vi "ActionVIOnCompile.vi"(8 "error in (no error)":errorcluster, 11 "Device Item Ref in":T1 format="%.0x") -> (0 "error out":errorcluster)   [LabVIEW 2015, in "Waveform-Processing-Custom-Device System Explorer.lvlib"]
uses:
  Waveform-Processing-Custom-Device System Explorer.lvlib
  <vilib>/NI VeriStand/Custom Device API/Custom Device API.lvlib
  <vilib>/NI/NIVS Inline Async API/_Data Access System Explorer/Data Access System Explorer.lvlib
  <vilib>/NI Veristand/Custom Device API/Data Reference.ctl
  <vilib>/NI Veristand/Custom Device API/Block Data Reference.ctl
  <vilib>/NI Veristand/Custom Device API/Waveform Data Reference.ctl
  Shared/CompiledSettings.ctl
  Shared/Waveform-Processing-Custom-Device Shared.lvlib
  Shared/Types/FG Action.ctl
  Shared/Running Average/Running Average.lvlib
  Shared/Single Point/SinglePoint.lvlib
  Shared/Constants.vi
  <vilib>/NI Veristand/Custom Device API/Set Item Property (Variant).vi
  <vilib>/NI Veristand/Custom Device API/Custom Device Item Ref.ctl
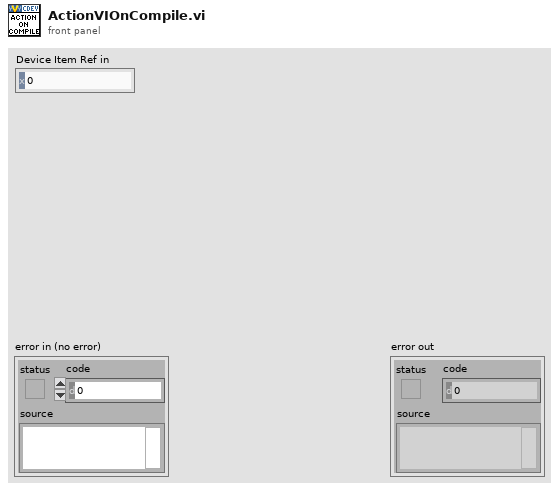
[diagram p1: front panel]
types:
  T1 = typedef "Custom Device API.lvlib/Custom Device Item Ref.ctl" = u64
  T2 = typedef "Waveform-Processing-Custom-Device Shared.lvlib/CompiledSettings.ctl" = cluster{"Name":string, "Buffer Length (samples)":u32, "Enable Array":bool[], "Parameter Block Data Refs":T3[], "Source Wfm Data Refs":T5[], "Result Wfm Data Refs":T5[], "Result Ch Data Refs":T4[], "Task Rate (Hz)":dbl}
  T3 = typedef "Custom Device API.lvlib/Block Data Reference.ctl" = cluster{"Data Reference":T4, "Offset":u64, "Length":u64}
  T4 = typedef "Custom Device API.lvlib/Data Reference.ctl" = i32
  T5 = typedef "Custom Device API.lvlib/Waveform Data Reference.ctl" = i32
  T6 = typedef "Waveform-Processing-Custom-Device Shared.lvlib/FG Action.ctl" = enum8{"GET", "SET"}
  T7 = typedef "Custom Device API.lvlib/Custom Device Item Info.ctl" = cluster{"Name":string, "Is Channel":bool, "GUID":string, "Is Waveform":bool}
  T8 = cluster{"Name":string, "Type":enum16{"Output/Write", "Input/Read", "Input/ReadWrite"}, "VS Refs":T1[]}[]
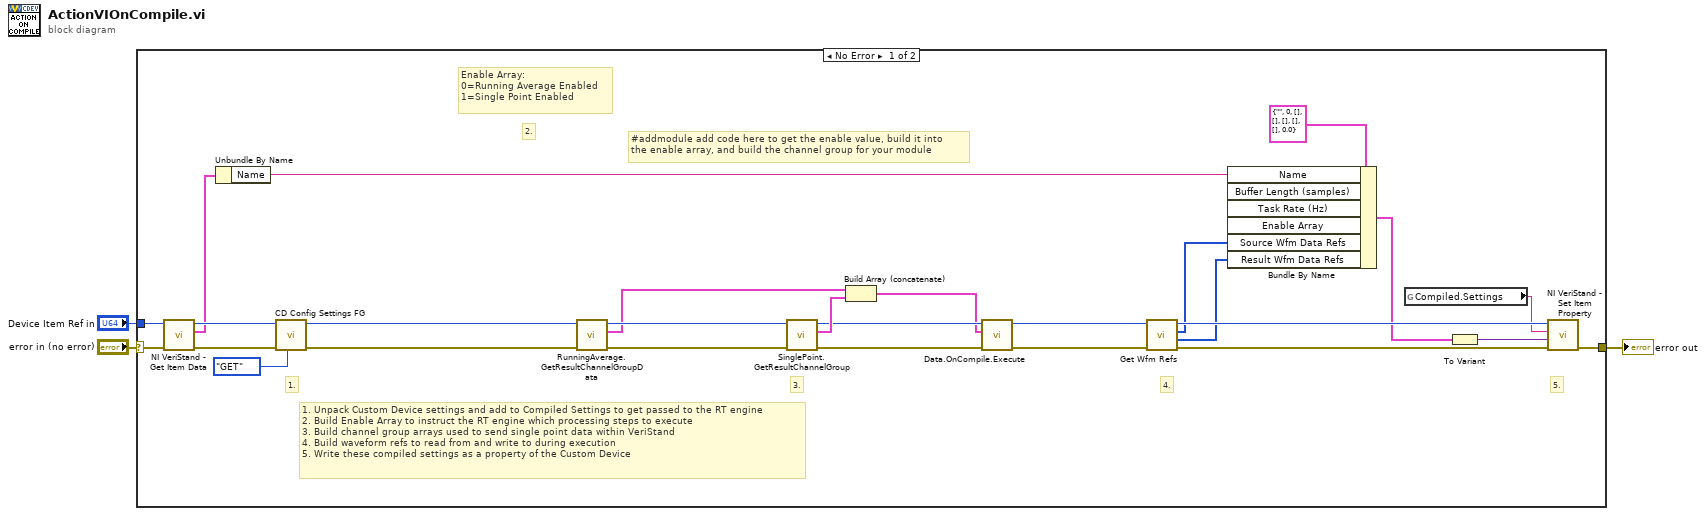
[diagram p0: block diagram]
diagram:
  n1 = case shown="No Error" "error in (no error)" {
    selector: "error in (no error)" -> [w29 w31]
    tunnel: [w30 w31] -> w2
    tunnel: "Device Item Ref in" -> [w28 _]
    frame No Error {
      # "#addmodule add code here to get the enable value, build it into\nthe enable array, and build the channel group for your module"
      # "Enable Array:\n0=Running Average Enabled\n1=Single Point Enabled"
      # "5."
      # "4."
      # "3."
      # "2."
      # "1."
      # "1. Unpack Custom Device settings and add to Compiled Settings to get passed to the RT engine\n2. Build Enable Array to instruct the RT engine which processing steps to execute\n3. Build channel group arrays used to send single point data within VeriStand\n4. Build waveform refs to read from and write to during execution\n5. Write these compiled settings as a property of the Custom Device"
      n2 = call <vilib>:"NI VeriStand - Get Item Data.vi"("error in (no error)"=w29, "Item Ref in"=w28) -> ("error out"=w26:errorcluster, "Item Info"=w25:T7, "Item Ref out"=w27:T1)  [unwired: 6 in, 1 out]
      n3 = Unbundle By Name(w25) -> ("Name"=w15:string)
      n4 = call "CD Config Settings FG.vi"("Action"=FG_Action."GET", "error in (no error)"=w26, "Item Ref"=w27) -> ("error out"=w23:errorcluster, "Item Ref out"=w18:T1)  [unwired: 5 in, 2 out]
      n5 = call "RunningAverage.GetResultChannelGroupData.vi"("Error in"=w23, "Device Ref in"=w18) -> ("Error out"=w22:errorcluster, "Group Data Array"=w14:T8, "Device Ref out"=w17:T1)  [unwired: 7 in]
      n6 = call "SinglePoint.GetResultChannelGroup.vi"("Error in"=w22, "Device Ref in"=w17) -> ("Error out"=w10:errorcluster, "Group Data Array"=w13:T8, "Device Ref out"=w12:T1)  [unwired: 7 in]
      n7 = Build Array (concatenate)(w14, w13) -> (w8:T8)
      n8 = call <vilib>:"Data.OnCompile.Execute.vi"("error in"=w10, "VS Ref Groups"=w8, "Custom Device Ref"=w12) -> ("error out"=w9:errorcluster, "Custom Device Ref"=w11:T1)  [unwired: 7 in]
      n9 = call "Get Wfm Refs.vi"("Error in"=w9, "Device Ref in"=w11) -> ("Error out"=w21:errorcluster, "Results Wfm Data Refs"=w6:T5[], "Source Wfm Data Refs"=w7:T5[], "Device Ref out"=w16:T1)  [unwired: 6 in]
      n10 = Bundle By Name(cluster=T2 {"Name"="", "Buffer Length (samples)"=0, "Enable Array"=[], "Parameter Block Data Refs"=[], "Source Wfm Data Refs"=[], "Result Wfm Data Refs"=[], "Result Ch Data Refs"=[], "Task Rate (Hz)"=0.0} ("CompiledSettings"), "Name"=w15, "Source Wfm Data Refs"=w7, "Result Wfm Data Refs"=w6) -> (w4:T2)  [unwired: 3 in]
      n11 = global read "Constants.vi" "Compiled.Settings"() -> (w5:string)
      n12 = To Variant(anything=w4) -> (Variant=w19:variant)
      n13 = call-poly <vilib>:"NI VeriStand - Set Item Property.vi"("error in (no error)"=w21, "Value"=w19, "Property Name"=w5, "Item Ref in"=w16) -> ("error out"=w30:errorcluster)  [unwired: 5 in, 2 out]
    }
    frame Error {
    }
  }
  "error out" <- w2
